vi "Write_output_file.vi"(0 "Output filename":path, 1 "Header":string, 2 "Template Filename":path, 5 "Channel Names":string[](array[string]), 7 "Data":string[][](array[string]), 9 "Desired Columns":i32[](array[numeric])=[0, 1, 2, 3, 4, 5, 6, 7, 8, 9, 10, 11, 12, 13, 14, 15, 16, 17, 18, 19, 20, 21, 22, 23, 24, 25, 26, 27, 28, 29, 30, 31, 32, 33, 34, 35, 36, 37, 38, 39, 40, 41, 42, 43, 44, 45, 46, 47, 48, 49, 50, 51, 52, 53, 54, 55, 56, 57, 58, 59, 60, 61, 62, 63, 64, 65, 66, 67, 68, 69, 70, 71, 72, 73, 74, 75, 76, 77, 78, 79, 80, 81, 82, 83, 84, 85, 86, 87, 88, 89, 90, 91, 92, 93, 94, 95, 96, 97, 98, 99, 100, 101, 102, 103, 104, 105, 106, 107, 108, 109, 110, 111, 112, 113, 114, 115, 116, 117, 118, 119, 120, 121, 122, 123, 124, 125, 126, 127, 128, 129, 130, 131, 132, 133, 134, 135, 136, 137, 138, 139, 140, 141, 142, 143, 144, 145, 146, 147, 148, 149, 150, 151, 152, 153, 154, 155, 156, 157, 158, 159, 160, 161, 162, 163, 164, 165, 166, 167, 168, 169, 170, 171, 172, 173, 174, 175, 176, 177, 178, 179, 180, 181, 182, 183, 184, 185, 186, 187, 188, 189, 190, 191, 192, 193, 194, 195, 196, 197, 198, 199, 200, 201, 202, 203, 204, 205, 206, 207, 208, 209, 210, 211, 212, 213, 214, 215, 216, 217, 218, 219, 220, 221, 222, 223, 224, 225, 226, 227, 228, 229, 230, 231, 232, 233, 234], 11 "Simple Save?":bool, 12 "Save Plotted rows only?":bool, 13 "Summarise mode":T2(ring), 14 "Grouping info":T3[](array[typedef]), 15 "Channels to Tabulate in header":i32[](listbox)) -> (4 "Output filename Out":path)   [LabVIEW 2010]
uses:
  Controls/Group_Binning.ctl
  Results_plotter_Global.vi
panel:
  out "Which Button?":T1(ring)=enum."Center Button"
  out "Table Values":string[][](array[string])
  out "Table Names":string[](array[string])
  out "Table":string
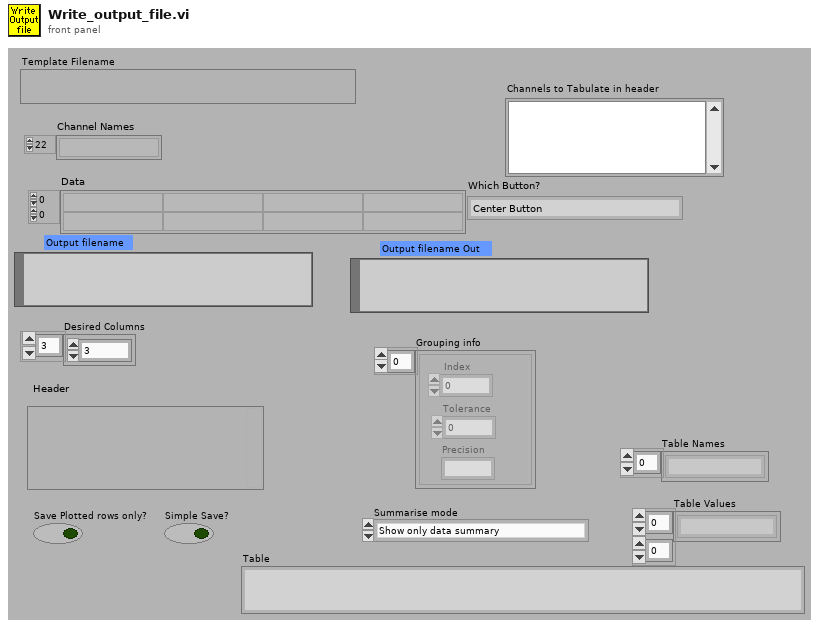
[diagram p1: front panel]
types:
  T1 = enum16{"Left Button", "Center Button", "Right Button", "Window Close"}
  T2 = enum16{"Show only data summary", "Show data summary", "No data summary"}
  T3 = typedef "Group_Binning.ctl" = cluster{"Index":i32, "Tolerance":dbl, "Precision":string}
  T4 = enum32{"existing file", "new file", "new or existing file", "existing dir", "new dir", "new or existing dir", "existing file (use LLBs)", "new file (use LLBs)", "new or existing file (use LLBs)", "new or existing file or directory (use LLBs)"}
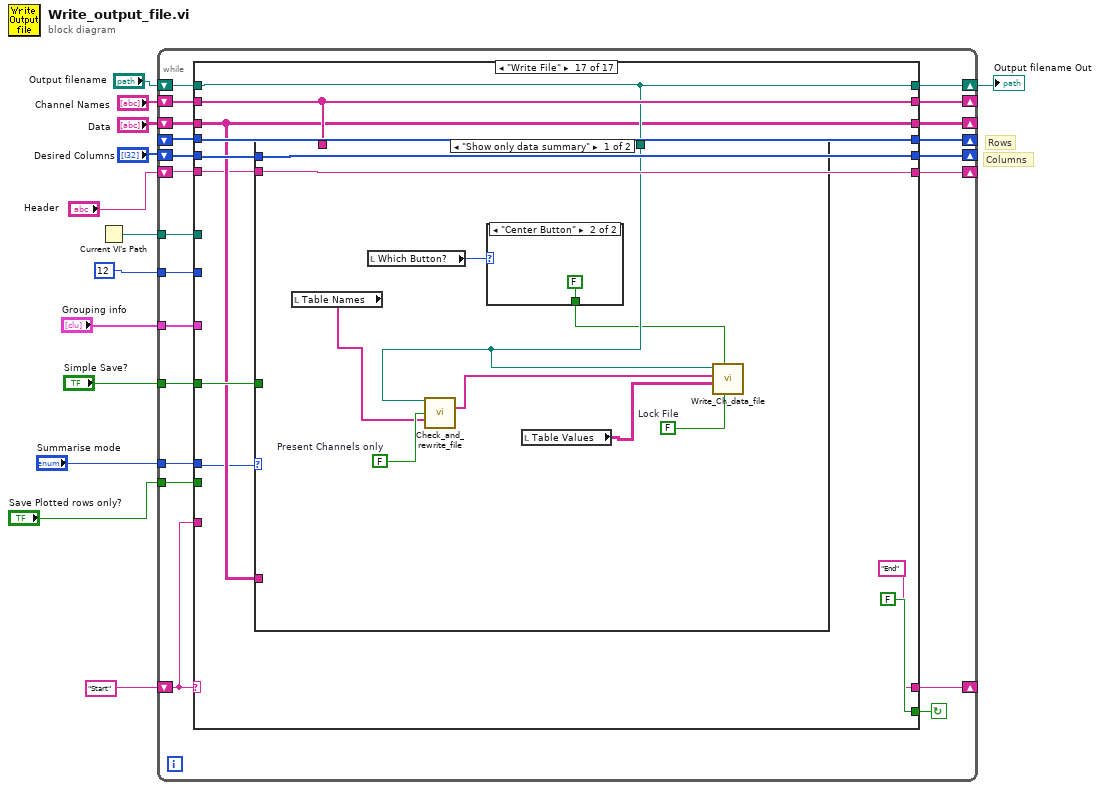
[diagram p0: block diagram]
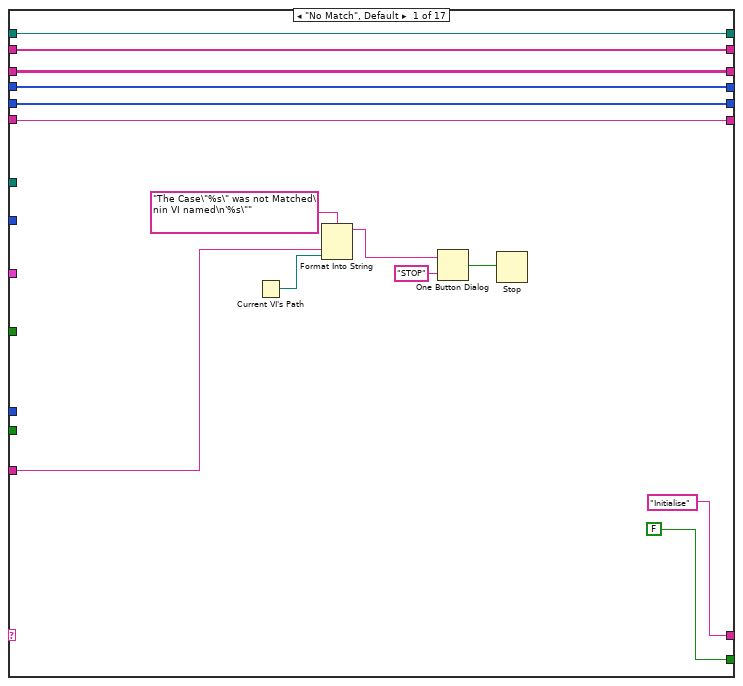
[diagram p2: hidden frame]
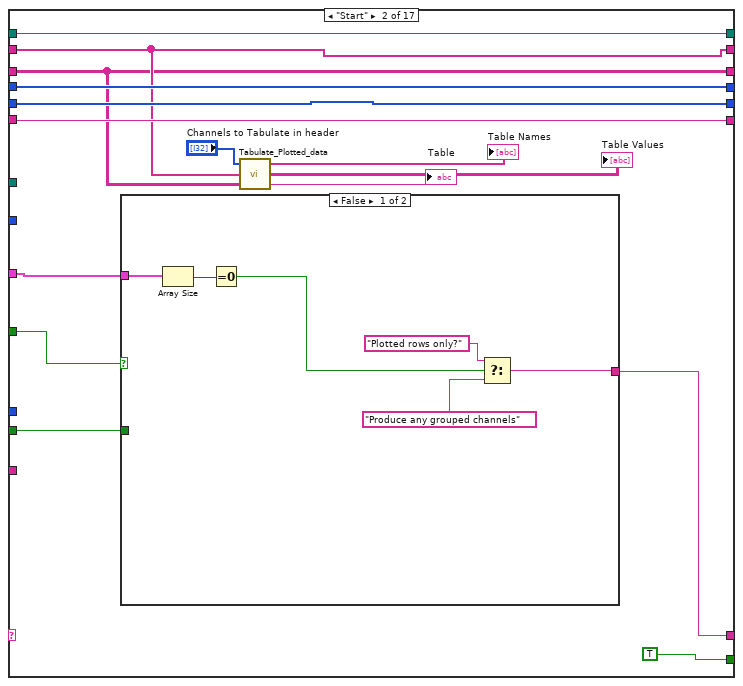
[diagram p3: hidden frame]
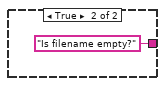
[diagram p4: hidden frame]
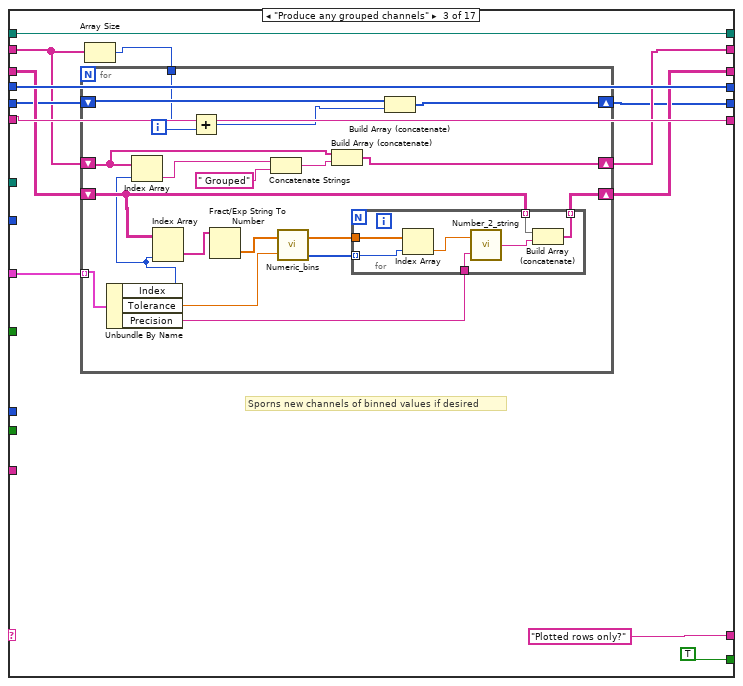
[diagram p5: hidden frame]
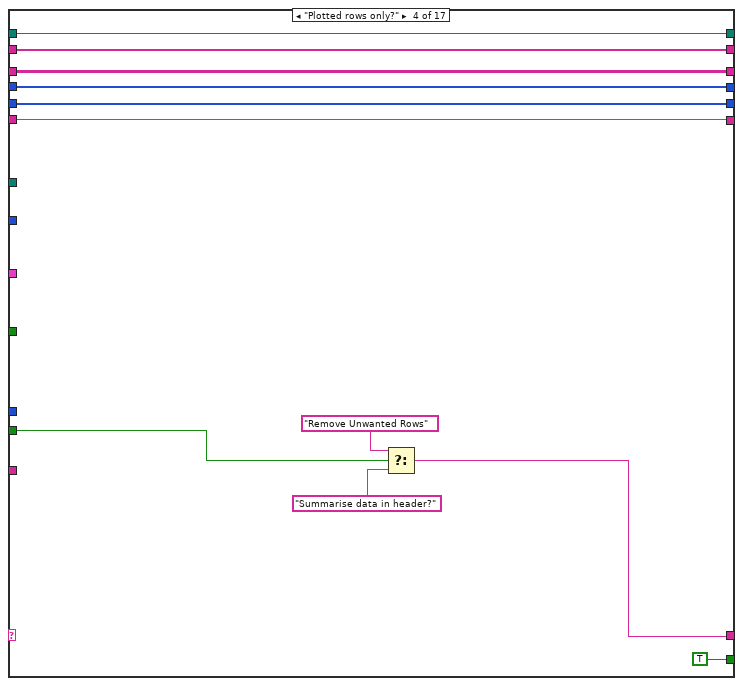
[diagram p6: hidden frame]
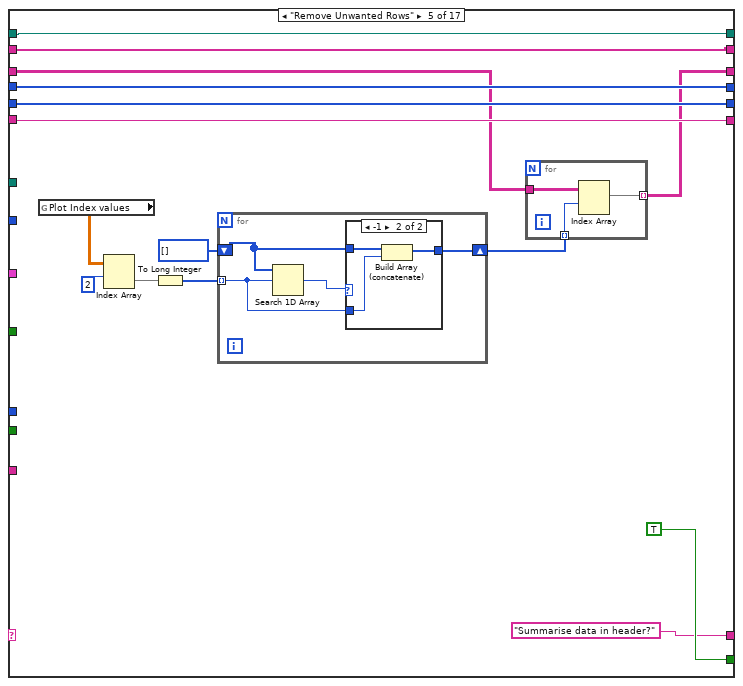
[diagram p7: hidden frame]
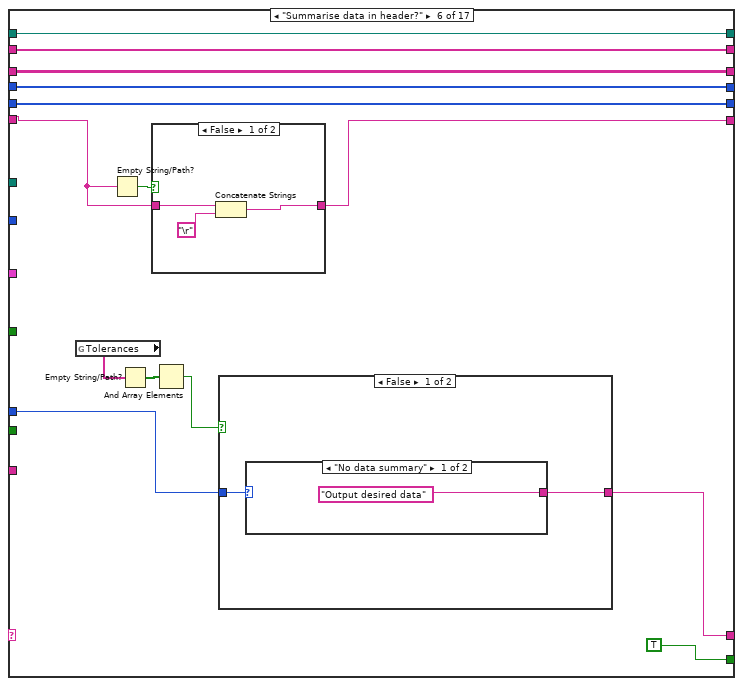
[diagram p9: hidden frame]
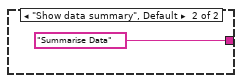
[diagram p10: hidden frame]
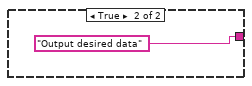
[diagram p11: hidden frame]
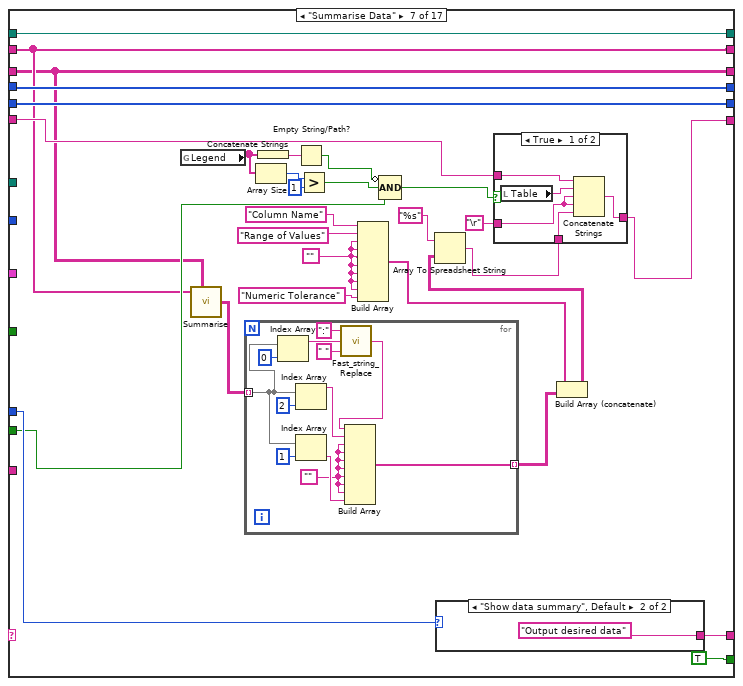
[diagram p13: hidden frame]
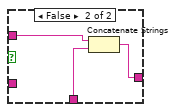
[diagram p14: hidden frame]
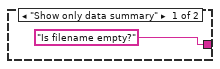
[diagram p15: hidden frame]
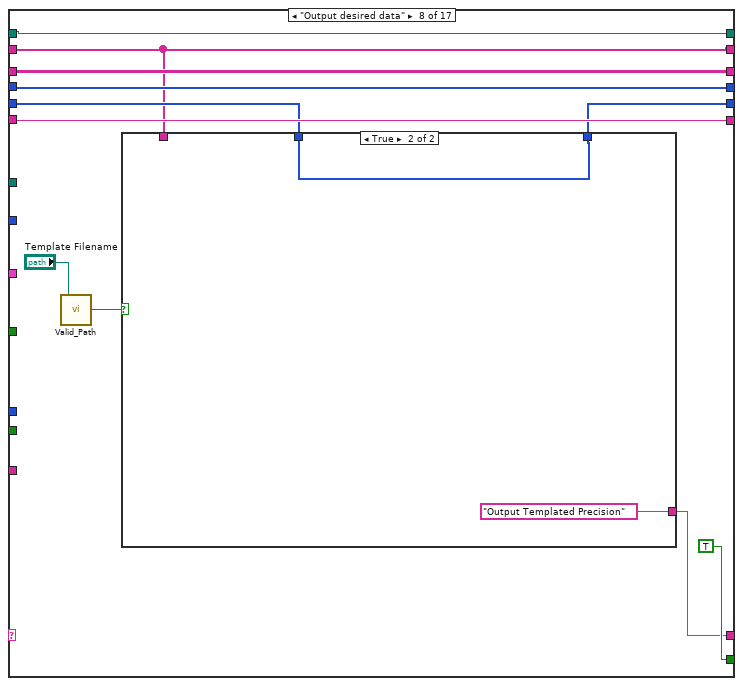
[diagram p16: hidden frame]
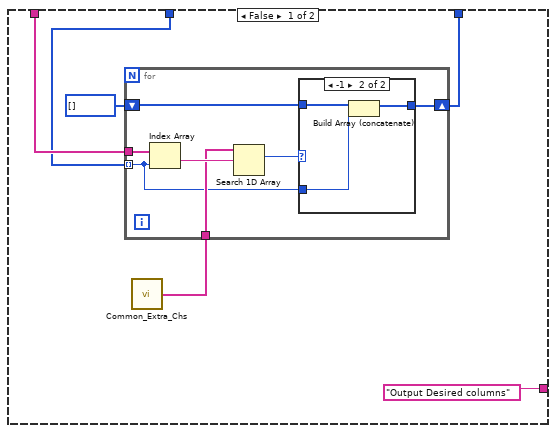
[diagram p17: hidden frame]
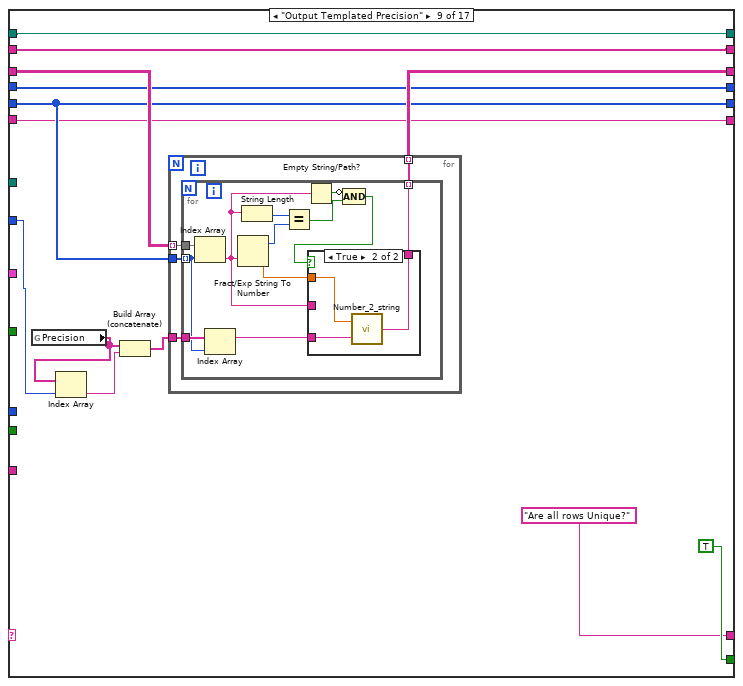
[diagram p19: hidden frame]
diagram:
  # "Columns"
  # "Rows"
  n1 = Current VI's Path() -> (path=w11:path)
  n2 = while {
    shift-left: "Header" -> [w24]
    shift-right: [w27] -> _
    shift-left: "Desired Columns" -> [w26]
    shift-right: [w25] -> _
    shift-left: _ -> [w28]
    shift-right: [w29] -> _
    shift-left: "Data" -> [w31]
    shift-right: [w30] -> _
    shift-left: "Start" -> [w32]
    shift-right: [w33] -> _
    tunnel: w11 -> [w23]
    shift-right: [w22] -> w10
    shift-left: "Output filename" -> [w21]
    shift-right: [w19] -> _
    shift-left: "Channel Names" -> [w20]
    tunnel: "Simple Save?" -> [w18]
    tunnel: 12 ("disabled index (col)") -> [w17]
    tunnel: "Grouping info" -> [w16]
    tunnel: "Summarise mode" -> [w15]
    tunnel: "Save Plotted rows only?" -> [w14]
    stop <- w34 continue-if-true
    n3 = case shown="\"Write File\"" w32 {
      tunnel: [FALSE TRUE TRUE TRUE ("cancelled") TRUE TRUE TRUE TRUE TRUE TRUE TRUE TRUE w358 w374 TRUE ("cancelled") FALSE ("cancelled") FALSE] -> w34
      tunnel: ["Initialise" w60 "Plotted rows only?" w112 "Summarise data in header?" w159 w195 w229 "Are all rows Unique?" "Is filename empty?" w305 "Is filename empty?" w359 w375 "Write File" "End" "End"] -> w33
      tunnel: w32 -> [w43 _ _ _ _ _ _ _ _ _ _ _ _ _ _ _ _]
      tunnel: w31 -> [w40 w53 w79 w116 w128 w155 w171 w226 w263 w292 w312 w348 w363 w385 w404 w418 w444]
      tunnel: [w40 w53 w77 w116 w127 w155 w171 w226 w262 w287 w312 w347 w363 w385 w404 w418 w444] -> w30
      tunnel: [w39 w62 w82 w115 w135 w160 w198 w231 w261 w291 w311 w346 w364 w386 w407 w427 w451] -> w29
      tunnel: w28 -> [w39 w62 w82 w115 w135 w160 w198 w231 w261 w291 _ w346 w364 w386 w407 w427 w451]
      tunnel: [w37 w61 w80 w113 w134 w151 w196 w230 w259 w289 w303 w343 w365 w387 w399 w428 w443] -> w27
      tunnel: w26 -> [w38 w57 w75 w114 w133 w154 w197 w228 w260 w290 w304 w344 w366 w388 w402 w409 w450]
      tunnel: [w38 w57 w72 w114 w133 w154 w197 w227 w260 w290 w304 w344 w366 w388 w402 w409 w450] -> w25
      tunnel: w24 -> [w37 w61 w80 w113 w134 w152 w173 w230 w259 w289 w303 w343 w365 w387 w397 w428 w443]
      tunnel: w23 -> [_ _ _ _ _ _ _ _ _ _ _ _ _ _ _ _ _]
      tunnel: [w36 w59 w81 w118 w123 w158 w194 w225 w257 w286 w302 w342 w362 w383 w401 w414 w446] -> w22
      tunnel: w21 -> [w36 w59 w81 w118 w123 w158 w194 w225 w257 w286 w302 w342 w355 w383 w401 w414 w446]
      tunnel: w20 -> [w35 w54 w74 w117 w122 w156 w172 w224 w256 w285 w301 w341 w357 w382 w403 w411 w447]
      tunnel: [w35 w54 w76 w117 w122 w156 w172 w224 w256 w285 w301 w341 w357 w382 w403 w411 w447] -> w19
      tunnel: w18 -> [_ w58 _ _ _ _ _ _ _ _ _ _ _ _ _ w410 w445]
      tunnel: w17 -> [_ _ _ _ _ _ _ _ w255 _ _ _ _ _ _ _ _]
      tunnel: w16 -> [_ w51 w78 _ _ _ _ _ _ _ _ _ _ _ _ _ _]
      tunnel: w15 -> [_ _ _ _ _ w157 w193 _ _ _ _ _ _ _ _ _ w442]
      tunnel: w14 -> [_ w56 _ w120 _ _ w192 _ _ _ _ _ _ _ _ _ _]
      frame "No Match", Default {
        n4 = Current VI's Path() -> (path=w42:path)
        n5 = Format Into String(format string="The Case\"%s\" was not Matched\nin VI named\n'%s\"" ("Format String"), w43, w42) -> (resulting string=w46:string)  [unwired: 2 in, 1 out]
        n6 = One Button Dialog(message=w46, button name ("OK")="STOP") -> (true=w44:bool)
        n7 = Stop(stop? (T)=w44) -> ()
      }
      frame "Start" {
        n8 = case shown="False" w58 {
          tunnel: [w64 "Is filename empty?" ("f")] -> w60
          tunnel: w56 -> [_ _]
          tunnel: w51 -> [w68 _]
          frame False {
            n9 = Array Size(array=w68) -> (size(s)=w69:i32)
            n10 = Equal To 0?(x=w69) -> (x = 0?=w67:bool)
            n11 = Select(t="Plotted rows only?", s=w67, f="Produce any grouped channels") -> (s? t:f=w64:string)
          }
          frame True {
          }
        }
        n12 = call "Tabulate_Plotted_data.vi"("Data"=w53, "Channel Names"=w54, "Channels to Tabulate"="Channels to Tabulate in header") -> ("spreadsheet string"=→"Table":string, "Channel Values"=→"Table Values":string[][], "Channel Names"=→"Table Names":string[])
      }
      frame "Produce any grouped channels" {
        # "Sporns new channels of binned values if desired"
        n13 = Array Size(array=w74) -> (size(s)=w73:i32)
        n14 = for {
          shift-right: [w95] -> w77
          shift-left: w79 -> [w96]
          tunnel: w78 -> [w100] mode=indexing
          shift-right: [w89] -> w76
          shift-left: w74 -> [w90]
          shift-right: [w87] -> w72
          shift-left: w75 -> [w88]
          tunnel: w73 -> [w85]
          i -> [w86]
          n15 = Unbundle By Name(w100) -> ("Index"=w94:i32, "Tolerance"=w98:dbl, "Precision"=w97:string)
          n16 = Index Array(array=w90, index=w94) -> (element=w92:string)
          n17 = Index Array(array=w96, index (col)=w94) -> (element=w99:string[])  [unwired: 1 in]
          n18 = Add(x=w85, y=w86) -> (x+y=w84:i32)
          n19 = Fract/Exp String To Number(string=w99) -> (number=w103:dbl[])  [unwired: 4 out]
          n20 = Concatenate Strings(w92, " Grouped" ("string")) -> (w91:string)
          n21 = call "Numeric_bins.vi"("Values"=w103, "Tolerance"=w98) -> ("Bin Centres"=w102:dbl[], "Bin Index"=w101:i32[])  [unwired: 1 out]
          n22 = Build Array (concatenate)(w90, w91) -> (w89:string[])
          n23 = for {
            tunnel: w102 -> [w110]
            tunnel: w101 -> [w109] mode=indexing
            tunnel: [w106] -> w95 mode=indexing
            tunnel: w97 -> [w105]
            tunnel: w96 -> [w104] mode=indexing
            n24 = Index Array(array=w110, index=w109) -> (element=w108:dbl)
            n25 = call "Number_2_string.vi"("precision"=w105, "number"=w108) -> ("String"=w107:string)
            n26 = Build Array (concatenate)(w104, w107) -> (w106:string[])
          }
          n27 = Build Array (concatenate)(w88, w84) -> (w87:i32[])
        }
      }
      frame "Plotted rows only?" {
        n28 = Select(t="Remove Unwanted Rows" ("f"), s=w120, f="Summarise data in header?") -> (s? t:f=w112:string)
      }
      frame "Remove Unwanted Rows" {
        n29 = global read "Results_plotter_Global.vi" "Plot Index values"() -> (w132:dbl[][])
        n30 = Index Array(array=w132, index (row)=2 ("disabled index (col)")) -> (element=w131:dbl[])  [unwired: 1 in]
        n31 = To Long Integer(number=w131) -> (32bit integer=w130:i32[])
        n32 = for {
          shift-right: [w141] -> w126
          shift-left: i32[] [] -> [w142]
          tunnel: w130 -> [w140] mode=indexing
          n33 = Search 1D Array(1D array=w142, element=w140) -> (index of element=w143:i32)  [unwired: 1 out]
          n34 = case shown="-1" w143 {
            tunnel: w142 -> [w144 w147]
            tunnel: [w144 w146] -> w141
            tunnel: w140 -> [_ w145]
            frame 0, Default {
            }
            frame -1 {
              n35 = Build Array (concatenate)(w147, w145) -> (w146:i32[])
            }
          }
        }
        n36 = for {
          tunnel: w126 -> [w139] mode=indexing
          tunnel: w128 -> [w138]
          tunnel: [w137] -> w127 mode=indexing
          n37 = Index Array(array=w138, index (row)=w139) -> (element=w137:string[])  [unwired: 1 in]
        }
      }
      frame "Summarise data in header?" {
        n38 = global read "Results_plotter_Global.vi" "Tolerances"() -> (w150:string[])
        n39 = Empty String/Path?(string/path=w152) -> (empty?=w153:bool)
        n40 = Empty String/Path?(string/path=w150) -> (empty?=w149:bool[])
        n41 = case shown="False" w153 {
          tunnel: [w167 w170] -> w151
          tunnel: w152 -> [w168 w170]
          frame False {
            n42 = Concatenate Strings(w168, "\r") -> (w167:string)
          }
          frame True {
          }
        }
        n43 = And Array Elements(Boolean array=w149) -> (logical AND=w148:bool)
        n44 = case shown="False" w148 {
          tunnel: [w163 "Output desired data" ("t")] -> w159
          tunnel: w157 -> [w162 _]
          frame False {
            n45 = case shown="\"No data summary\"" w162 {
              tunnel: ["Output desired data" ("t") "Summarise Data"] -> w163
              frame "No data summary" {
              }
              frame "Show data summary", Default {
              }
            }
          }
          frame True {
          }
        }
      }
      frame "Summarise Data" {
        w183 = ""
        n46 = global read "Results_plotter_Global.vi" "Legend"() -> (w180:string[])
        n47 = call "Summarise.vi"("Channel Names"=w172, "Data"=w171) -> ("Summary"=w190:string[][])  [unwired: 2 in, 1 out]
        n48 = for {
          tunnel: w190 -> [w216] mode=indexing
          tunnel: [w208] -> w174 mode=indexing
          w209 = ""
          n49 = Index Array(array=w216, index=0) -> (element=w213:string)
          n50 = Index Array(array=w216, index=2) -> (element=w214:string)
          n51 = Index Array(array=w216, index=1) -> (element=w215:string)
          n52 = call "Fast_string_Replace.vi"("Replace match with:"=" ", "Input String"=w213, "regular expression"=":") -> ("Output String"=w210:string)  [unwired: 2 out]
          n53 = Build Array(w210, w214, w209, w209, w209, w209, w209, w209, w209, w215) -> (w208:string[])
        }
        n54 = Array Size(array=w180) -> (size(s)=w178:i32)
        n55 = Concatenate Strings(w180) -> (w182:string)
        n56 = Empty String/Path?(string/path=w182) -> (empty?=w176:bool)
        n57 = Greater?(x=w178, y=1) -> (0:w175:bool)
        n58 = Build Array("Column Name", "Range of Values", w183, w183, w183, w183, w183, w183, w183, "Numeric Tolerance") -> (w189:string[])
        n59 = Compound Arithmetic op=AND(invert w176, w175, w192) -> (w181:bool)
        n60 = case shown="\"Show data summary\", Default" w193 {
          tunnel: ["Is filename empty?" "Output desired data"] -> w195
          frame "Show only data summary" {
          }
          frame "Show data summary", Default {
          }
        }
        n61 = Build Array (concatenate)(w189, w174) -> (w188:string[][])
        n62 = Array To Spreadsheet String(array=w188, 3:"%s" ("format string")) -> (spreadsheet string=w185:string)  [unwired: 1 out]
        n63 = case shown="True" w181 {
          tunnel: [w201 w206] -> w196
          tunnel: w173 -> [w204 w205]
          tunnel: w185 -> [w202 w207]
          tunnel: "\r" -> [w203 _]
          frame True {
            n64 = local read "Table"() -> (w200:string)
            n65 = Concatenate Strings(w204, w200, w203, w203, w202) -> (w201:string)
          }
          frame False {
            n66 = Concatenate Strings(w205, w207) -> (w206:string)
          }
        }
      }
      frame "Output desired data" {
        n67 = call "Valid_Path.vi"("Filename"="Template Filename") -> ("Valid Path?"=w222:bool)
        n68 = case shown="True" w222 {
          tunnel: ["Output Desired columns" "Output Templated Precision" ("f")] -> w229
          tunnel: w228 -> [w236 w250]
          tunnel: [w234 w250] -> w227
          tunnel: w224 -> [w237 _]
          frame False {
            n69 = call "Common_Extra_Chs.vi"() -> ("Common Extra Channels"=w233:string[])
            n70 = for {
              shift-right: [w239] -> w234
              shift-left: i32[] [] -> [w241]
              tunnel: w237 -> [w245]
              tunnel: w236 -> [w240] mode=indexing
              tunnel: w233 -> [w243]
              n71 = Index Array(array=w245, index=w240) -> (element=w244:string)
              n72 = Search 1D Array(1D array=w243, element=w244) -> (index of element=w242:i32)  [unwired: 1 out]
              n73 = case shown="-1" w242 {
                tunnel: w241 -> [w246 w249]
                tunnel: w240 -> [_ w248]
                tunnel: [w246 w247] -> w239
                frame 0, Default {
                }
                frame -1 {
                  n74 = Build Array (concatenate)(w249, w248) -> (w247:i32[])
                }
              }
            }
          }
          frame True {
          }
        }
      }
      frame "Output Templated Precision" {
        n75 = global read "Results_plotter_Global.vi" "Precision"() -> (w254:string[])
        n76 = Index Array(array=w254, index=w255) -> (element=w252:string)
        n77 = Build Array (concatenate)(w254, w252) -> (w253:string[])
        n78 = for {
          tunnel: w260 -> [w268]
          tunnel: w263 -> [w267] mode=indexing
          tunnel: w253 -> [w266]
          tunnel: [w265] -> w262 mode=indexing
          n79 = for {
            tunnel: w268 -> [w278] mode=indexing
            tunnel: w267 -> [w280]
            tunnel: w266 -> [w279]
            tunnel: [w272] -> w265 mode=indexing
            n80 = Index Array(array=w280, index=w278) -> (element=w271:string)
            n81 = Index Array(array=w279, index=w278) -> (element=w270:string)
            n82 = Fract/Exp String To Number(string=w271) -> (offset past number=w276:i32, number=w273:dbl)  [unwired: 3 out]
            n83 = String Length(string=w271) -> (length=w277:i32)
            n84 = Equal?(x=w277, y=w276) -> (x = y?=w274:bool)
            n85 = Empty String/Path?(string/path=w271) -> (empty?=w275:bool)
            n86 = Compound Arithmetic op=AND(invert w275, w274) -> (w269:bool)
            n87 = case shown="True" w269 {
              tunnel: w270 -> [_ w283]
              tunnel: w273 -> [_ w284]
              tunnel: [w281 w282] -> w272
              tunnel: w271 -> [w281 _]
              frame False {
              }
              frame True {
                n88 = call "Number_2_string.vi"("precision"=w283, "number"=w284) -> ("String"=w282:string)
              }
            }
          }
        }
      }
      frame "Output Desired columns" {
        n89 = for {
          tunnel: w290 -> [w296]
          tunnel: w292 -> [w295] mode=indexing
          tunnel: [w294] -> w287 mode=indexing
          n90 = for {
            tunnel: w296 -> [w298] mode=indexing
            tunnel: w295 -> [w299]
            tunnel: [w297] -> w294 mode=indexing
            n91 = Index Array(array=w299, index=w298) -> (element=w297:string)
          }
        }
      }
      frame "Are all rows Unique?" {
        n92 = for {
          shift-right: [w318] -> _
          shift-left: _ -> [w317]
          tunnel: w312 -> [w320] mode=indexing
          shift-right: [w316] -> w311
          shift-left: _ -> [w315]
          tunnel: [w314] -> w308
          i -> [w314]
          n93 = Array To Spreadsheet String(array=w320, 3:"%s" ("format string")) -> (spreadsheet string=w319:string)  [unwired: 1 out]
          n94 = case shown="0" w314 {
            tunnel: w319 -> [w325 w331]
            tunnel: [w324 w328] -> w318
            tunnel: w317 -> [_ w332]
            tunnel: [w322 w329] -> w316
            tunnel: w315 -> [_ w330]
            tunnel: w314 -> [_ w326]
            frame 0 {
              n95 = Build Array(w325) -> (w324:string[])
              n96 = Build Array(0) -> (w322:i32[])
            }
            frame 1, Default {
              n97 = Search 1D Array(1D array=w332, element=w331) -> (index of element=w327:i32)  [unwired: 1 out]
              n98 = case shown="-1" w327 {
                tunnel: w332 -> [w334 w340]
                tunnel: w331 -> [_ w339]
                tunnel: w330 -> [w333 w338]
                tunnel: [w333 w337] -> w329
                tunnel: [w334 w336] -> w328
                tunnel: w326 -> [_ w335]
                frame 0, Default {
                }
                frame -1 {
                  n99 = Build Array (concatenate)(w340, w339) -> (w336:string[])
                  n100 = Build Array (concatenate)(w338, w335) -> (w337:i32[])
                }
              }
            }
          }
        }
        n101 = Array Size(array=w311) -> (size(s)=w310:i32)
        n102 = Decrement(x=w310) -> (x-1=w309:i32)
        n103 = Equal?(x=w309, y=w308) -> (x = y?=w300:bool)
        n104 = Select(t="Is filename empty?", s=w300, f="Remove Duplicate Rows") -> (s? t:f=w305:string)
      }
      frame "Remove Duplicate Rows" {
        n105 = for {
          tunnel: w346 -> [w352] mode=indexing
          tunnel: w348 -> [w351]
          tunnel: [w350] -> w347 mode=indexing
          n106 = Index Array(array=w351, index (row)=w352) -> (element=w350:string[])  [unwired: 1 in]
        }
      }
      frame "Is filename empty?" {
        n107 = call "Append_Suffiix.vi"("Results file"=w355) -> ("appended path"=w354:path)
        n108 = call "Valid_Path.vi"("Filename"=w354) -> ("Valid Path?"=w356:bool)
        n109 = case shown="False" w356 {
          tunnel: [w367 w373] -> w362
          tunnel: w354 -> [_ w373]
          tunnel: [w369 TRUE ("cancelled")] -> w358
          frame False {
            (unwired) T4."new or existing file" ("select mode (2)")
            n110 = File Dialog(7:"Save Output file as:" ("prompt")) -> (1:w370:bool, 3:w368:path)  [unwired: 1 in, 7 out]
            n111 = Not(x=w370) -> (.not. x?=w369:bool)
            n112 = call "Append_Suffiix.vi"("Results file"=w368) -> ("appended path"=w367:path)
          }
          frame True {
          }
        }
        n113 = call "Does_file_exist_(simple).vi"("Pathname"=w362) -> ("exists?"=w361:bool)
        n114 = Select(t="Check for overwrite or append", s=w361, f="Write File") -> (s? t:f=w359:string)
      }
      frame "Check for overwrite or append" {
        n115 = Format Into String(format string="Do you want to append to the result file\n\"%s\"" ("message"), w383) -> (resulting string=w380:string)  [unwired: 2 in, 1 out]
        n116 = call <vilib>:"Three Button Dialog.vi"("Window Title (\"\")"="Output File Dialog" ("Window Title (\"\")"), "Right Button Text (\"Cancel\")"="Cancel" ("Button 3 Name"), "Center Button Text (\"No\")"="Overwrite" ("F button name (\"Cancel\")"), "Left Button Text (\"Yes\")"="Append" ("T button name (\"OK\")"), "message"=w380) -> ("Which Button?"=w381:T1)  [unwired: 6 out]
        "Which Button?" <- w381
        n117 = case shown="\"Right Button\"" w381 {
          tunnel: ["Append to Results file" ("t") "Write File" "End" ("t") "End"] -> w375
          tunnel: [TRUE TRUE FALSE FALSE] -> w374
          frame "Left Button" {
          }
          frame "Center Button" {
          }
          frame "Right Button" {
          }
          frame "Window Close" {
          }
        }
      }
      frame "Append to Results file" {
        w398 = "\r"
        n118 = call "Read_File_Simple.vi"("Filename"=w401) -> ("string"=w400:string)  [unwired: 2 in, 7 out]
        n119 = Concatenate Strings(w400, w398, w398, w398, w397) -> (w399:string)
      }
      frame "Append and Merge Results file" {
        w415 = TRUE  # Read Channel Names only
        w417 = FALSE  # Append last row only
        w421 = TRUE  # exists?
        w424 = FALSE  # Present Channels only
        n120 = case shown="False" w410 {
          tunnel: w409 -> [w431 _]
          tunnel: w411 -> [w430 w435]
          tunnel: [w429 w435] -> w408
          frame False {
            n121 = for {
              tunnel: w431 -> [w432] mode=indexing
              tunnel: w430 -> [w434]
              tunnel: [w433] -> w429 mode=indexing
              n122 = Index Array(array=w434, index=w432) -> (element=w433:string)
            }
          }
          frame True {
          }
        }
        n123 = call "Read_Data_file.vi"("Results file"=w414, "Read Channel Names only"=w415, "Template File"=path "") -> ("String Before"=w413:string)  [unwired: 2 in, 14 out]
        n124 = String Length(string=w413) -> (length=w412:i32)
        n125 = call "Check_and_rewrite_file.vi"("Filename"=w414, "Present Channels only"=w424, "Present Channels"=w408, "Start of read offset (chars.: 0)"=w412) -> ("Merged Channels"=w423:string[], "Merged?"=w422:bool)  [unwired: 10 out]
        n126 = case shown="False" w422 {
          tunnel: [w437 w439] -> w420
          tunnel: w408 -> [w437 w441]
          tunnel: w418 -> [w436 w440]
          tunnel: [w436 w438] -> w419
          tunnel: w423 -> [_ w439]
          frame False {
          }
          frame True {
            n127 = call "Merge_2D_values.vi"("Values In"=w440, "Present Channels"=w441, "Desired Channels"=w439) -> ("Values Out"=w438:string[][])
          }
        }
        n128 = call "Write_Ch_data_file.vi"("Append last row only"=w417, "Header string"=w413, "exists?"=w421, "Channel Values"=w419, "Channel names"=w420, "Filename"=w414) -> ()  [unwired: 2 in, 4 out]
      }
      frame "Write File" {
        n129 = case shown="\"Show only data summary\"" w442 {
          tunnel: w450 -> [_ w474]
          tunnel: w447 -> [_ w473]
          tunnel: w446 -> [w456 w471]
          tunnel: w445 -> [_ w468]
          tunnel: w444 -> [_ w466]
          tunnel: w443 -> [_ w464]
          frame "Show only data summary" {
            w457 = FALSE  # Present Channels only
            w459 = FALSE  # Lock File
            n130 = local read "Table Names"() -> (w455:string[])
            n131 = local read "Which Button?"() -> (w453:T1)
            n132 = call "Check_and_rewrite_file.vi"("Filename"=w456, "Present Channels only"=w457, "Present Channels"=w455) -> ("Merged Channels"=w458:string[])  [unwired: 1 in, 11 out]
            n133 = case shown="\"Center Button\"" w453 {
              tunnel: [w460 FALSE ("exists?")] -> w452
              frame "Left Button", Default {
                w460 = TRUE  # exists?
              }
              frame "Center Button" {
              }
            }
            n134 = local read "Table Values"() -> (w454:string[][])
            n135 = call "Write_Ch_data_file.vi"("Lock File"=w459, "exists?"=w452, "Channel Values"=w454, "Channel names"=w458, "Filename"=w456) -> ()  [unwired: 3 in, 4 out]
          }
          frame "Show data summary", Default {
            w470 = FALSE  # Append last row only
            w472 = FALSE  # exists?
            n136 = global read "Results_plotter_Global.vi" "Description"() -> (w462:string[])
            n137 = Empty String/Path?(string/path=w464) -> (empty?=w463:bool)
            n138 = case shown="True" w468 {
              tunnel: w474 -> [w481 _]
              tunnel: w462 -> [w480 _]
              tunnel: [w476 w487] -> w465
              tunnel: w473 -> [w479 w488]
              tunnel: [w478 w488] -> w467
              tunnel: w466 -> [w475 w487]
              frame False {
                n139 = for {
                  tunnel: w481 -> [w483] mode=indexing
                  tunnel: w479 -> [w486]
                  tunnel: [w485] -> w478 mode=indexing
                  tunnel: w480 -> [w484]
                  tunnel: [w482] -> w477 mode=indexing
                  n140 = Index Array(array=w486, index=w483) -> (element=w485:string)
                  n141 = Index Array(array=w484, index=w483) -> (element=w482:string)
                }
                n142 = Build Array (concatenate)(w477, w475) -> (w476:string[][])
              }
              frame True {
              }
            }
            n143 = case shown="False" w463 {
              tunnel: [w491 ""] -> w469
              tunnel: w464 -> [w489 _]
              frame False {
                n144 = Initialize Array("", 10 ("Dimension Size")) -> (w494:string[])
                n145 = call "Asterisk_header.vi"("Channel names"=w494) -> ("Header string"=w493:string)
                n146 = Concatenate Strings(w489, "\r", "#" ("Substring"), w493) -> (w491:string)
              }
              frame True {
              }
            }
            n147 = call "Write_Ch_data_file.vi"("Append last row only"=w470, "Header string"=w469, "exists?"=w472, "Channel Values"=w465, "Channel names"=w467, "Filename"=w471) -> ()  [unwired: 2 in, 4 out]
          }
        }
      }
    }
  }
  "Output filename Out" <- w10
